vi "Order JointState By Name.vi"(0 "Ordered Joint Names":string[](array[string]), 2 "JointState In":T1) -> (7 "JointState Out":T1)   [LabVIEW 2013]
uses:
  labview_msgs/sensor_msgs/JointState.ctl
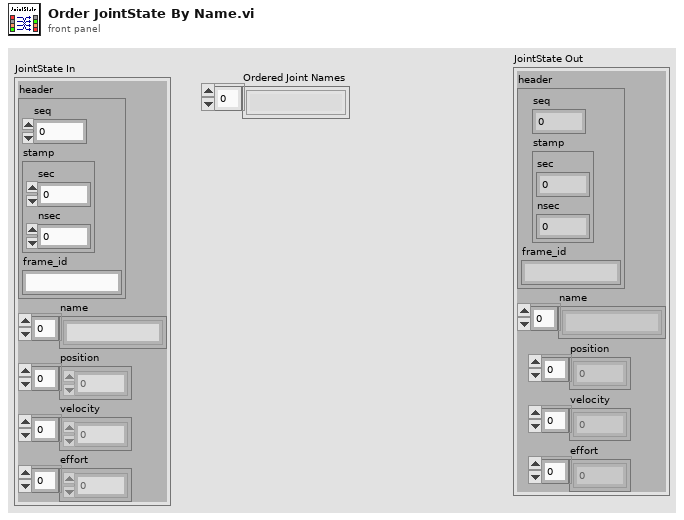
[diagram p1: front panel]
types:
  T1 = typedef "JointState.ctl" = cluster{"header":cluster{"seq":u32, "stamp":cluster{"sec":i32, "nsec":i32}, "frame_id":string}, "name":string[], "position":dbl[], "velocity":dbl[], "effort":dbl[]}
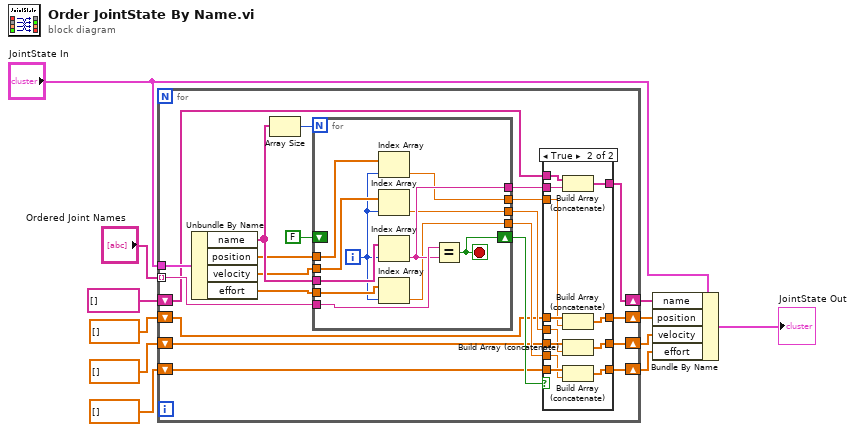
[diagram p0: block diagram]
diagram:
  n1 = for {
    tunnel: "JointState In" -> [w32]
    tunnel: "Ordered Joint Names" -> [w29] mode=indexing
    shift-right: [w13] -> w3
    shift-left: dbl[] [] -> [w12]
    shift-right: [w15] -> w4
    shift-left: dbl[] [] -> [w14]
    shift-right: [w17] -> w5
    shift-left: dbl[] [] -> [w16]
    shift-right: [w19] -> w6
    shift-left: string[] [] -> [w18]
    n2 = Unbundle By Name(w32) -> ("name"=w30:string[], "position"=w28:dbl[], "velocity"=w27:dbl[], "effort"=w26:dbl[])
    n3 = Array Size(array=w30) -> (size(s)=w31:i32)
    n4 = for {
      N: w31 -> [_]
      tunnel: w30 -> [w59]
      tunnel: w29 -> [w58]
      tunnel: w28 -> [w57]
      tunnel: w27 -> [w56]
      tunnel: w26 -> [w55]
      tunnel: [w53] -> w23
      tunnel: [w52] -> w22
      tunnel: [w51] -> w21
      tunnel: [w50] -> w20
      shift-right: [w49] -> w24
      shift-left: FALSE -> [_]
      i -> [w54]
      stop <- w49 stop-if-true
      n5 = Index Array(array=w57, index=w54) -> (element=w52:dbl)
      n6 = Index Array(array=w56, index=w54) -> (element=w51:dbl)
      n7 = Index Array(array=w59, index=w54) -> (element=w53:string)
      n8 = Index Array(array=w55, index=w54) -> (element=w50:dbl)
      n9 = Equal?(x=w58, y=w53) -> (x = y?=w49:bool)
    }
    n10 = case shown="True" w24 {
      tunnel: w23 -> [_ w46]
      tunnel: w22 -> [_ w43]
      tunnel: w21 -> [_ w40]
      tunnel: w20 -> [_ w37]
      tunnel: [w36 w48] -> w19
      tunnel: w18 -> [w36 w47]
      tunnel: [w35 w45] -> w17
      tunnel: w16 -> [w35 w44]
      tunnel: [w34 w42] -> w15
      tunnel: w14 -> [w34 w41]
      tunnel: [w33 w39] -> w13
      tunnel: w12 -> [w33 w38]
      frame False {
      }
      frame True {
        n11 = Build Array (concatenate)(w47, w46) -> (w48:string[])
        n12 = Build Array (concatenate)(w44, w43) -> (w45:dbl[])
        n13 = Build Array (concatenate)(w41, w40) -> (w42:dbl[])
        n14 = Build Array (concatenate)(w38, w37) -> (w39:dbl[])
      }
    }
  }
  n15 = Bundle By Name(cluster="JointState In", "name"=w6, "position"=w5, "velocity"=w4, "effort"=w3) -> (→"JointState Out":T1)
